vi "Write Offset Past Match.vi"(8 "error in (no error)":errorcluster, 10 "Abs_I32 Integer.lvclass":refnum<class "Abs_I32 Integer.lvclass">, 11 "MatchPattern_STR in":refnum<class "MatchPattern_STR.lvclass">) -> (0 "error out":errorcluster, 3 "MatchPattern_STR out":refnum<class "MatchPattern_STR.lvclass">)   [LabVIEW 2021, in "MatchPattern_STR.lvclass"]
uses:
  MatchPattern_STR.lvclass
  Abs_Types/I32 Integer/Abs_I32 Integer.lvclass
  MatchPattern_STR.lvclass/MatchPattern_STR.ctl
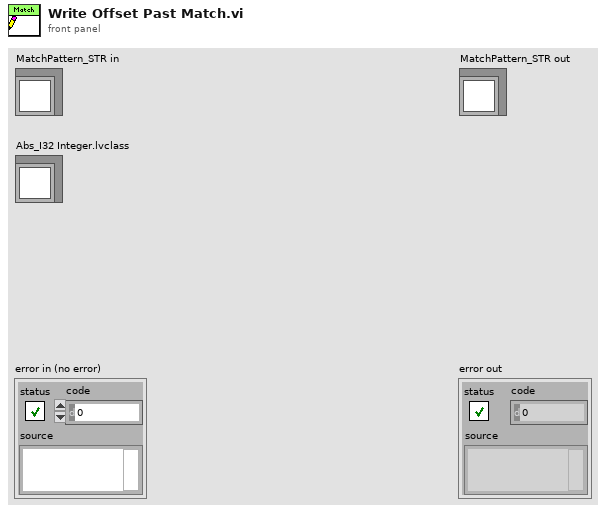
[diagram p1: front panel]
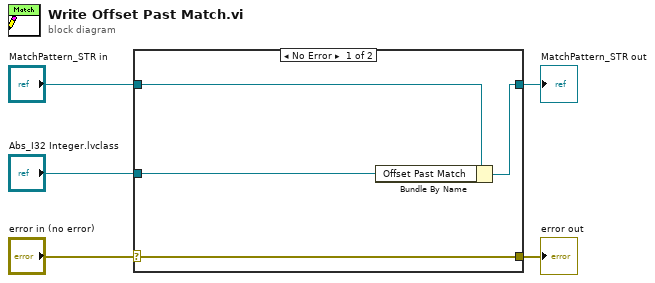
[diagram p0: block diagram]
diagram:
  n1 = case shown="No Error" "error in (no error)" {
    selector: "error in (no error)" -> [w9 w10]
    tunnel: [w9 w10] -> w4
    tunnel: [w7 w11] -> w2
    tunnel: "MatchPattern_STR in" -> [w8 w11]
    tunnel: "Abs_I32 Integer.lvclass" -> [w6 _]
    frame No Error {
      n2 = Bundle By Name(cluster=w8, "Offset Past Match"=w6) -> (w7:refnum<class "MatchPattern_STR.lvclass">)
    }
    frame Error {
    }
  }
  "error out" <- w4
  "MatchPattern_STR out" <- w2
